vi "tsdb_load_can_db_win32.vi"(8 "错误输入（无错误）":errorcluster, 10 "ASupportedChannelsBased0":string, 11 "路径":path) -> (0 "错误输出":errorcluster, 2 "out AId":u32, 3 "tsdb_load_can_db":i32)   [LabVIEW 2016]
uses:
  TSMaster.dll
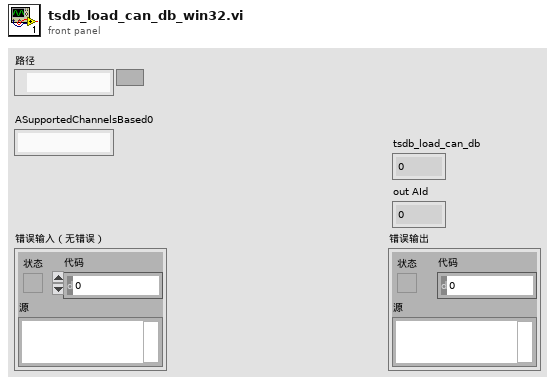
[diagram p1: front panel]
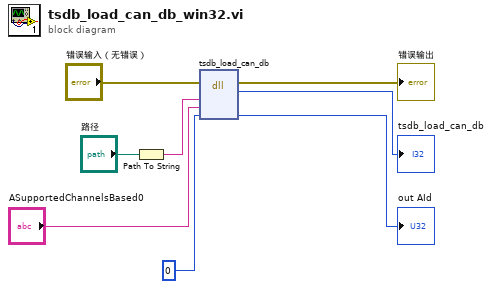
[diagram p0: block diagram]
diagram:
  n1 = Path To String(path="路径") -> (string=w3:string)
  n2 = dll-call lib="C:/Users/Eric/Desktop/LabVIEW/TSMasterAPI/Win32/TSMaster_LV2010_Release/TSMaster.dll" fn="tsdb_load_can_db"(error in="错误输入（无错误）", "ADBC"=w3, "ASupportedChannelsBased0"="ASupportedChannelsBased0", "out AId"=u32 0) -> (error out=→"错误输出":errorcluster, "tsdb_load_can_db"=→"tsdb_load_can_db":i32, "out AId"=→"out AId":u32)  [unwired: 4 in, 1 out]
